vi "SRTS_Save.vi"(8 "error in":errorcluster, 10 "DAQ data":T1, 11 "TDMS in":refnum<class "TDMS.lvclass">) -> (0 "error out":errorcluster, 3 "TDMS out":refnum<class "TDMS.lvclass">)   [LabVIEW 2017, in "Report_lib.lvlib" / "TDMS.lvclass"]
uses:
  TDMS.lvclass
  TypeDefs/DAQ data.ctl
  TDMS.lvclass/TDMS.ctl
  Channels names.ctl
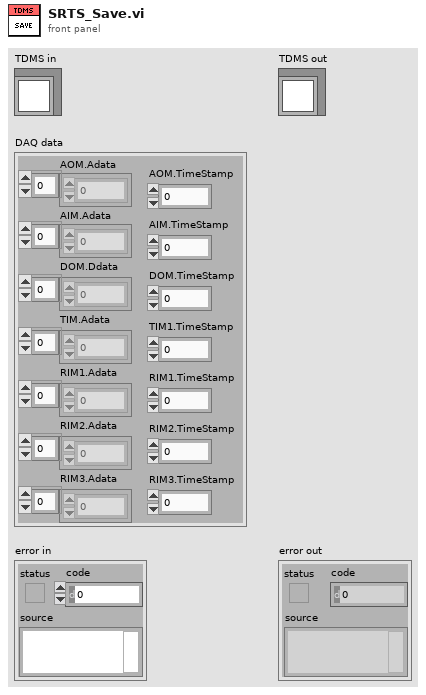
[diagram p1: front panel]
types:
  T1 = typedef "DAQ data.ctl" = cluster{"AOM.Adata":dbl[], "AIM.Adata":dbl[], "RIM1.Adata":dbl[], "TIM.Adata":dbl[], "RIM2.Adata":dbl[], "RIM3.Adata":dbl[], "DOM.Ddata":dbl[], "AOM.TimeStamp":dbl, "AIM.TimeStamp":dbl, "DOM.TimeStamp":dbl, "TIM1.TimeStamp":dbl, "RIM1.TimeStamp":dbl, "RIM2.TimeStamp":dbl, "RIM3.TimeStamp":dbl}
  T2 = typedef "Channels names.ctl" = cluster{"AIM ch.names":string[], "TIM ch.names":string[], "RIM1 ch.names":string[], "RIM2 ch.names":string[], "RIM3 ch.names":string[], "AOM ch.names":string[], "DOM ch.hames":string[]}
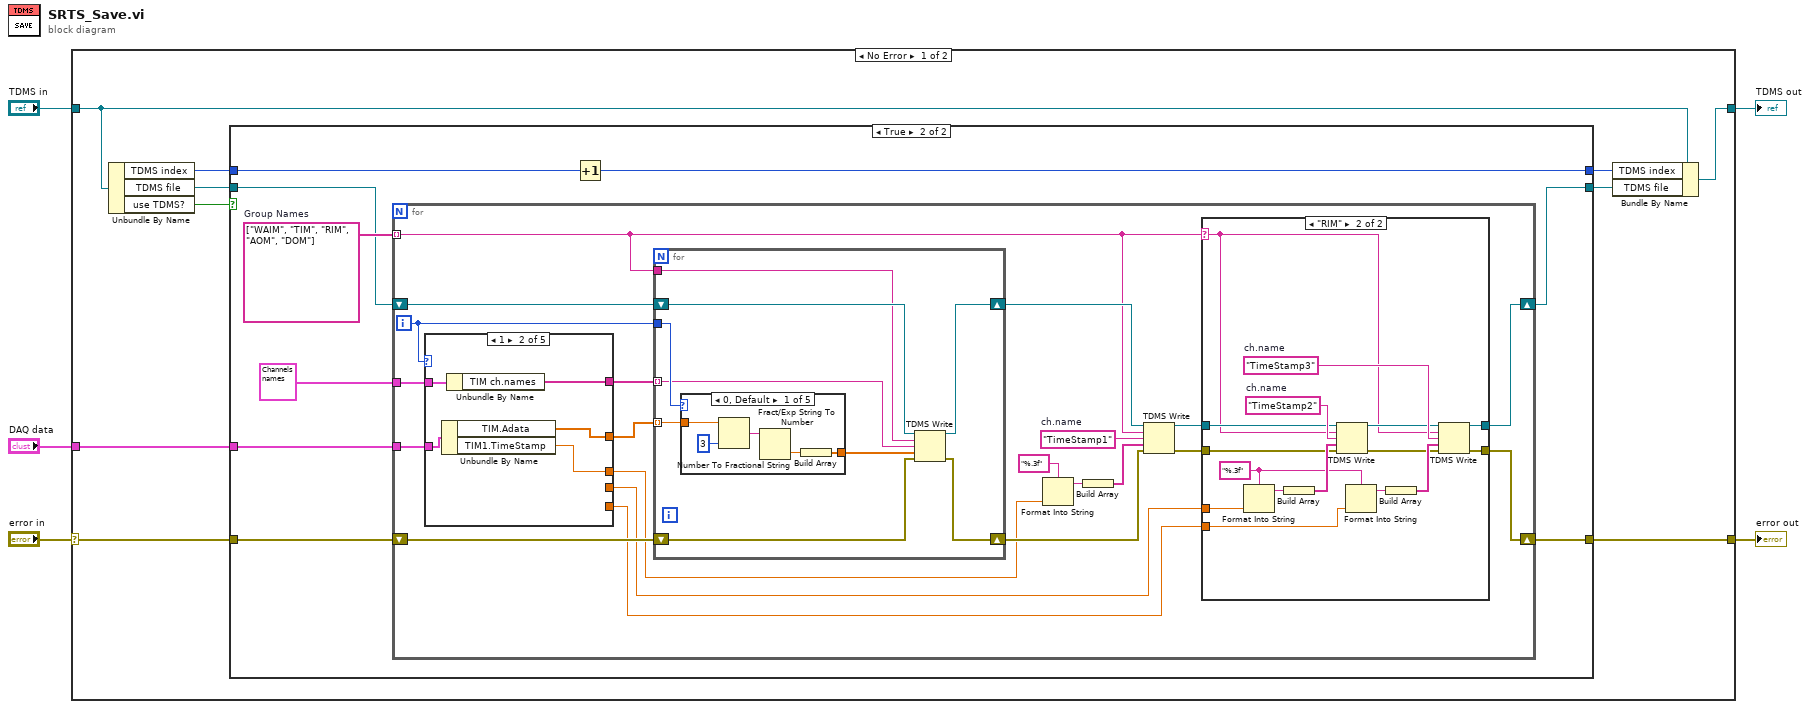
[diagram p0: block diagram]
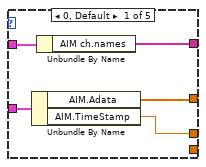
[diagram p4: hidden frame]
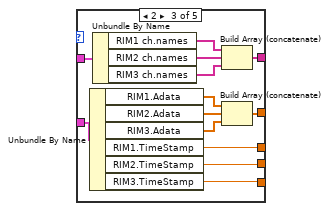
[diagram p5: hidden frame]
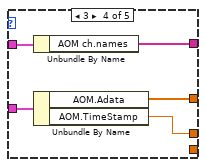
[diagram p6: hidden frame]
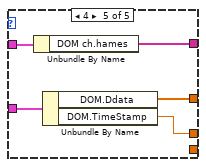
[diagram p7: hidden frame]
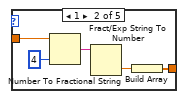
[diagram p8: hidden frame]
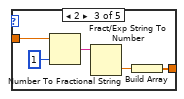
[diagram p9: hidden frame]
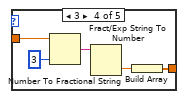
[diagram p10: hidden frame]
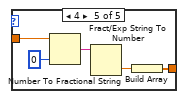
[diagram p11: hidden frame]
diagram:
  n1 = case shown="No Error" "error in" {
    selector: "error in" -> [w14 w135]
    tunnel: [w7 w135] -> w1
    tunnel: [w9 w134] -> w3
    tunnel: "TDMS in" -> [w10 w134]
    tunnel: "DAQ data" -> [w8 _]
    frame No Error {
      n2 = Unbundle By Name(w10) -> ("TDMS index"=w13:i32, "TDMS file"=w15:refnum<k34>, "use TDMS?"=w6:bool)
      n3 = case shown="True" w6 {
        tunnel: w15 -> [w17 w26]
        tunnel: w14 -> [w16 w25]
        tunnel: w13 -> [w18 w24]
        tunnel: [w18 w23] -> w12
        tunnel: [w17 w22] -> w11
        tunnel: w8 -> [_ w21]
        tunnel: [w16 w20] -> w7
        frame False {
        }
        frame True {
          w27 = string[] ["WAIM", "TIM", "RIM", "AOM", "DOM"]  # Group Names
          n4 = for {
            tunnel: w27 -> [w34] mode=indexing
            tunnel: T2 {"AIM ch.names"=["05_waim_01ch", "05_waim_02ch", "05_waim_03ch", "05_waim_04ch", "05_waim_05ch", "05_waim_06ch", "05_waim_07ch", "05_waim_08ch", "05_waim_09ch", "05_waim_10ch", "05_waim_11ch", "05_waim_12ch", "05_waim_13ch", "05_waim_14ch", "05_waim_15ch", "05_waim_16ch", "05_waim_17ch", "05_waim_18ch", "05_waim_19ch", "05_waim_20ch", "05_waim_21ch", "05_waim_22ch", "05_waim_23ch", "05_waim_24ch", "05_waim_25ch", "05_waim_26ch", "05_waim_27ch", "05_waim_28ch", "05_waim_29ch", "05_waim_30ch", "05_waim_31ch", "05_waim_32ch", "01_tim_17ch", "01_tim_18ch", "01_tim_19ch", "01_tim_20ch", "01_tim_21ch", "01_tim_22ch", "01_tim_23ch", "01_tim_24ch", "01_tim_25ch", "01_tim_26ch", "01_tim_27ch", "01_tim_28ch", "01_tim_29ch", "01_tim_30ch", "01_tim_31ch", "01_tim_32ch"], "TIM ch.names"=["01_tim_01ch", "01_tim_02,14:16ch", "01_tim_03:09ch", "01_tim_10:13ch"], "RIM1 ch.names"=["02_rim_01ch", "02_rim_02ch", "02_rim_03ch", "02_rim_04ch", "02_rim_05ch", "02_rim_06ch", "02_rim_07ch", "02_rim_08ch", "reserve1"], "RIM2 ch.names"=["03_rim_01ch", "03_rim_02ch", "03_rim_03ch", "03_rim_04ch", "03_rim_05ch", "03_rim_06ch", "03_rim_07ch", "03_rim_08ch", "reserve2"], "RIM3 ch.names"=["04_rim_01ch", "04_rim_02ch", "04_rim_03ch", "04_rim_04ch", "04_rim_05ch", "04_rim_06ch", "04_rim_07ch", "04_rim_08ch", "reserve3"], "AOM ch.names"=["05_aom_01ch", "05_aom_02ch", "05_aom_03ch", "05_aom_04ch", "05_aom_05ch", "05_aom_06ch", "05_aom_07ch", "05_aom_08ch", "05_aom_09ch", "05_aom_10ch", "05_aom_11ch", "05_aom_12ch", "05_aom_13ch", "05_aom_14ch", "05_aom_15ch", "05_aom_16ch", "05_aom_17ch", "05_aom_18ch", "05_aom_19ch", "05_aom_20ch", "05_aom_21ch", "05_aom_22ch", "05_aom_23ch", "05_aom_24ch"], "DOM ch.hames"=["03_dom_01ch", "03_dom_02ch", "03_dom_03ch", "03_dom_04ch", "03_dom_05ch", "03_dom_06ch", "03_dom_07ch", "03_dom_08ch", "03_dom_09ch", "03_dom_10ch", "03_dom_11ch", "03_dom_12ch", "03_dom_13ch", "03_dom_14ch", "03_dom_15ch", "03_dom_16ch", "03_dom_17ch", "03_dom_18ch", "03_dom_19ch", "03_dom_20ch", "03_dom_21ch", "03_dom_22ch", "03_dom_23ch", "03_dom_24ch"]} ("Modules Channels names") -> [w47]
            tunnel: w21 -> [w48]
            shift-right: [w30] -> w22
            shift-left: w26 -> [w43]
            shift-right: [w31] -> w20
            shift-left: w25 -> [w42]
            i -> [w44]
            w41 = "TimeStamp1"  # ch.name
            n5 = case shown="1" w44 {
              tunnel: w48 -> [w71 w76 w89 w94 w99]
              tunnel: w47 -> [w70 w75 w88 w93 w98]
              tunnel: [w69 w74 w80 w92 w97] -> w46
              tunnel: [w68 w72 w84 w91 w96] -> w45
              tunnel: [w67 w73 w79 w90 w95] -> w36
              tunnel: [_ _ w78 _ _] -> w29
              tunnel: [_ _ w77 _ _] -> w28
              frame 0, Default {
                n6 = Unbundle By Name(w71) -> ("AIM.Adata"=w69:dbl[], "AIM.TimeStamp"=w67:dbl)
                n7 = Unbundle By Name(w70) -> ("AIM ch.names"=w68:string[])
              }
              frame 1 {
                n8 = Unbundle By Name(w76) -> ("TIM.Adata"=w74:dbl[], "TIM1.TimeStamp"=w73:dbl)
                n9 = Unbundle By Name(w75) -> ("TIM ch.names"=w72:string[])
              }
              frame 2 {
                n10 = Unbundle By Name(w89) -> ("RIM1.Adata"=w81:dbl[], "RIM2.Adata"=w82:dbl[], "RIM3.Adata"=w83:dbl[], "RIM1.TimeStamp"=w79:dbl, "RIM2.TimeStamp"=w78:dbl, "RIM3.TimeStamp"=w77:dbl)
                n11 = Unbundle By Name(w88) -> ("RIM1 ch.names"=w87:string[], "RIM2 ch.names"=w86:string[], "RIM3 ch.names"=w85:string[])
                n12 = Build Array (concatenate)(w87, w86, w85) -> (w84:string[])
                n13 = Build Array (concatenate)(w81, w82, w83) -> (w80:dbl[])
              }
              frame 3 {
                n14 = Unbundle By Name(w93) -> ("AOM ch.names"=w91:string[])
                n15 = Unbundle By Name(w94) -> ("AOM.Adata"=w92:dbl[], "AOM.TimeStamp"=w90:dbl)
              }
              frame 4 {
                n16 = Unbundle By Name(w98) -> ("DOM ch.hames"=w96:string[])
                n17 = Unbundle By Name(w99) -> ("DOM.Ddata"=w97:dbl[], "DOM.TimeStamp"=w95:dbl)
              }
            }
            n18 = for {
              tunnel: w46 -> [w107] mode=indexing
              tunnel: w45 -> [w104] mode=indexing
              tunnel: w44 -> [w108]
              shift-right: [w105] -> w38
              shift-left: w43 -> [w106]
              tunnel: w34 -> [w103]
              shift-right: [w100] -> w39
              shift-left: w42 -> [w101]
              n19 = case shown="0, Default" w108 {
                tunnel: w107 -> [w110 w115 w120 w125 w130]
                tunnel: [w109 w114 w119 w124 w129] -> w102
                frame 0, Default {
                  n20 = Number To Fractional String(number=w110, precision (6)=i16 3) -> (F-format string=w112:string)  [unwired: 2 in]
                  n21 = Fract/Exp String To Number(string=w112) -> (number=w113:dbl)  [unwired: 3 in, 1 out]
                  n22 = Build Array(w113) -> (w109:dbl[])
                }
                frame 1 {
                  n23 = Number To Fractional String(number=w115, precision (6)=i16 4) -> (F-format string=w117:string)  [unwired: 2 in]
                  n24 = Fract/Exp String To Number(string=w117) -> (number=w118:dbl)  [unwired: 3 in, 1 out]
                  n25 = Build Array(w118) -> (w114:dbl[])
                }
                frame 2 {
                  n26 = Number To Fractional String(number=w120, precision (6)=i16 1) -> (F-format string=w122:string)  [unwired: 2 in]
                  n27 = Fract/Exp String To Number(string=w122) -> (number=w123:dbl)  [unwired: 3 in, 1 out]
                  n28 = Build Array(w123) -> (w119:dbl[])
                }
                frame 3 {
                  n29 = Number To Fractional String(number=w125, precision (6)=i16 3) -> (F-format string=w127:string)  [unwired: 2 in]
                  n30 = Fract/Exp String To Number(string=w127) -> (number=w128:dbl)  [unwired: 3 in, 1 out]
                  n31 = Build Array(w128) -> (w124:dbl[])
                }
                frame 4 {
                  n32 = Number To Fractional String(number=w130, precision (6)=i16 0) -> (F-format string=w132:string)  [unwired: 2 in]
                  n33 = Fract/Exp String To Number(string=w132) -> (number=w133:dbl)  [unwired: 3 in, 1 out]
                  n34 = Build Array(w133) -> (w129:dbl[])
                }
              }
              n35 = TDMS Write(0:w106, 5:w103, 7:w104, 9:w102, 11:w101) -> (4:w105:refnum<k34>, 15:w100:errorcluster)  [unwired: 1 in, 2 out]
            }
            n36 = Format Into String(format string="%.3f", w36) -> (resulting string=w35:string)  [unwired: 2 in, 1 out]
            n37 = Build Array(w35) -> (w40:string[])
            n38 = TDMS Write(0:w38, 5:w34, 7:w41, 9:w40, 11:w39) -> (4:w33:refnum<k34>, 15:w32:errorcluster)  [unwired: 1 in, 2 out]
            n39 = case shown="\"RIM\"" w34 {
              selector: w34 -> [_ w54]
              tunnel: w33 -> [w49 w63]
              tunnel: w32 -> [w50 w62]
              tunnel: [w50 w55] -> w31
              tunnel: [w49 w56] -> w30
              tunnel: w29 -> [_ w53]
              tunnel: w28 -> [_ w52]
              frame Default {
              }
              frame "RIM" {
                w61 = "TimeStamp3"  # ch.name
                w51 = "%.3f" ("format string")
                w64 = "TimeStamp2"  # ch.name
                n40 = Format Into String(format string=w51, w53) -> (resulting string=w66:string)  [unwired: 2 in, 1 out]
                n41 = Build Array(w66) -> (w65:string[])
                n42 = TDMS Write(0:w63, 5:w54, 7:w64, 9:w65, 11:w62) -> (4:w58:refnum<k34>, 15:w57:errorcluster)  [unwired: 1 in, 2 out]
                n43 = Format Into String(format string=w51, w52) -> (resulting string=w59:string)  [unwired: 2 in, 1 out]
                n44 = Build Array(w59) -> (w60:string[])
                n45 = TDMS Write(0:w58, 5:w54, 7:w61, 9:w60, 11:w57) -> (4:w56:refnum<k34>, 15:w55:errorcluster)  [unwired: 1 in, 2 out]
              }
            }
          }
          n46 = Increment(x=w24) -> (x+1=w23:i32)
        }
      }
      n47 = Bundle By Name(cluster=w10, "TDMS index"=w12, "TDMS file"=w11) -> (w9:refnum<class "TDMS.lvclass">)
    }
    frame Error {
    }
  }
  "error out" <- w1
  "TDMS out" <- w3
